vi "Store Graph.vi"(5 "file (use dialog)":path=path "E:/LCU6331 test/printer/WEEE.PCX") -> (0 "read string":string, 2 "Stored successful?":bool)   [LabVIEW 2009]
uses:
  Global/Global 1.vi
panel:
  out "match substring":string
  out "file name":string
  out "size (in bytes)":i64
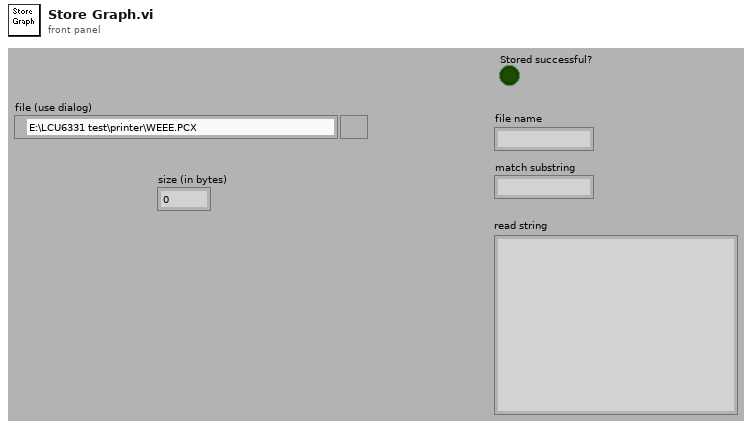
[diagram p1: front panel]
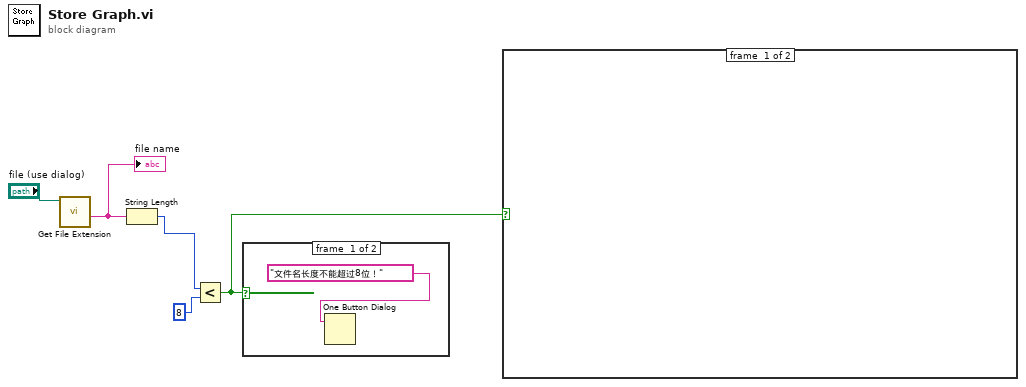
[diagram p0: block diagram]
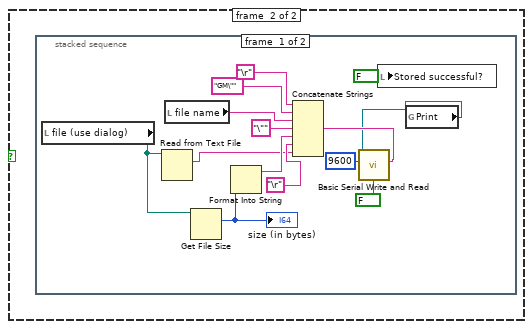
[diagram p3: hidden frame]
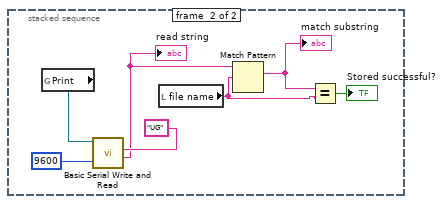
[diagram p4: hidden frame]
diagram:
  n1 = call <vilib>:"Get File Extension.vi"("file"="file (use dialog)") -> ("filename without extension"=w2:string)  [unwired: 1 in, 9 out]
  "file name" <- w2
  n2 = String Length(string=w2) -> (length=w4:i32)
  n3 = Less?(x=w4, y=8) -> (x < y?=w1:bool)
  n4 = case shown="False" w1 {
    frame #0 {
      n5 = One Button Dialog(message="文件名长度不能超过8位！") -> ()  [unwired: 2 out]
    }
    frame #1 {
    }
  }
  n6 = case shown="True" w1 {
    frame #0 {
    }
    frame #1 {
      n7 = stacked-sequence {
        frame #0 {
          n8 = local read "file (use dialog)"() -> (w17:path)
          n9 = Read from Text File(file (use dialog)=w17) -> (text=w13:string)  [unwired: 1 in, 5 out]
          n10 = local read "file name"() -> (w12:string)
          n11 = Get File Size(file=w17) -> (size (in bytes)=w16:i64)  [unwired: 1 in, 2 out]
          "size (in bytes)" <- w16
          n12 = Format Into String(w16) -> (resulting string=w15:string)  [unwired: 3 in, 1 out]
          n13 = Concatenate Strings("\r", "GM\"" ("string"), w12, "\"" ("string"), w15, "\r", w13) -> (w10:string)
          n14 = local write "Stored successful?"(FALSE ("Stored successful?")) -> ()
          n15 = global read "Global 1.vi" "Print"() -> (w7:refnum<visa-resource-name>)
          n16 = call "Basic Serial Write and Read.vi"("VISA resource name"=w7, "baud rate"=u32 9600, "read"=FALSE, "string to write"=w10) -> ()  [unwired: 5 in, 2 out]
        }
        frame #1 {
          n17 = global read "Global 1.vi" "Print"() -> (w21:refnum<visa-resource-name>)
          n18 = call "Basic Serial Write and Read.vi"("VISA resource name"=w21, "baud rate"=u32 9600, "string to write"="UG") -> ("read string"=w23:string)  [unwired: 6 in, 1 out]
          "read string" <- w23
          n19 = local read "file name"() -> (w26:string)
          n20 = Match Pattern(string=w23, regular expression=w26) -> (match substring=w27:string)  [unwired: 4 out]
          "match substring" <- w27
          n21 = Equal?(x=w27, y=w26) -> (x = y?=→"Stored successful?":bool)
        }
      }
    }
  }
